vi "Wrap Coordinates.vi"(10 "length":i32, 11 "index":i32=-1) -> (3 "translated index":i32)   [LabVIEW 2021, in "Game of Life.lvlib"]
doc: "This VI wraps the coordinates as below:\n-1 --> n-1\nn --> 0"
uses:
  Game of Life.lvlib
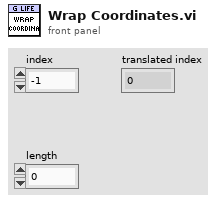
[diagram p1: front panel]
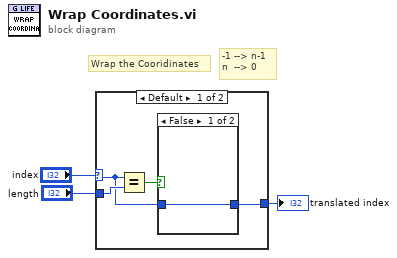
[diagram p0: block diagram]
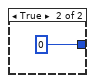
[diagram p2: hidden frame]
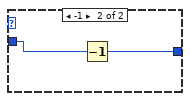
[diagram p3: hidden frame]
diagram:
  # "Wrap the Cooridinates"
  # "-1 --> n-1\nn  --> 0"
  n1 = case shown="Default" "index" {
    selector: "index" -> [w4 _]
    tunnel: "length" -> [w6 w11]
    tunnel: [w5 w10] -> w1
    frame Default {
      n2 = Equal?(x=w4, y=w6) -> (x = y?=w7:bool)
      n3 = case shown="False" w7 {
        tunnel: [w8 0 ("Column")] -> w5
        tunnel: w4 -> [w8 _]
        frame False {
        }
        frame True {
        }
      }
    }
    frame -1 {
      n4 = Decrement(x=w11) -> (x-1=w10:i32)
    }
  }
  "translated index" <- w1
